vi "RichToFlathwval_StatusResponse.vi"(5 "OutputClusterType":T1, 11 "InputCluster":T2) -> (3 "OutputCluster":T1)   [LabVIEW 2025, in "Automotive-Vision-OOBService_client.lvlib"]
uses:
  Automotive-Vision-OOBService_client.lvlib
  hwval_StatusResponse.ctl
  hwval_StatusResponse_Flat.ctl
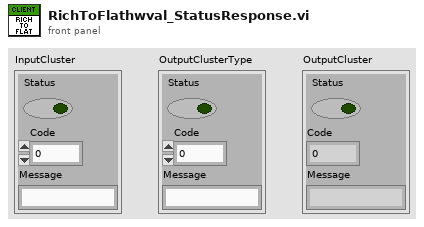
[diagram p1: front panel]
types:
  T1 = typedef "Automotive-Vision-OOBService_client.lvlib/hwval_StatusResponse_Flat.ctl" = cluster{"Status":bool, "Code":i32, "Message":string}
  T2 = typedef "Automotive-Vision-OOBService_client.lvlib/hwval_StatusResponse.ctl" = cluster{"Status":bool, "Code":i32, "Message":string}
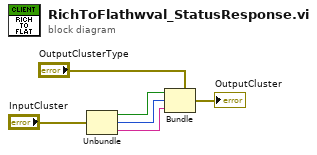
[diagram p0: block diagram]
diagram:
  n1 = Unbundle "Unbundle"("InputCluster") -> ("Status"=w3:bool, "Code"=w2:i32, "Message"=w1:string)
  n2 = Bundle "Bundle"(cluster="OutputClusterType", "Status"=w3, "Code"=w2, "Message"=w1) -> (→"OutputCluster":T1)
